vi "CalculateDatagram.vi"(0 "mqttCmd in":refnum<class "BaseMqttMsg.lvclass">, 5 "FixedHeaderByte1":u8 format="%08b", 7 "variableHeader":u8[](array[numeric]), 9 "payload":u8[](array[numeric]), 11 "error in (no error)":errorcluster) -> (4 "mqttCmd out":refnum<class "BaseMqttMsg.lvclass">, 6 "Datagram":u8[](array[numeric]), 15 "error out":errorcluster)   [LabVIEW 2020, in "BaseMqttMsg.lvclass"]
uses:
  BaseMqttMsg.lvclass
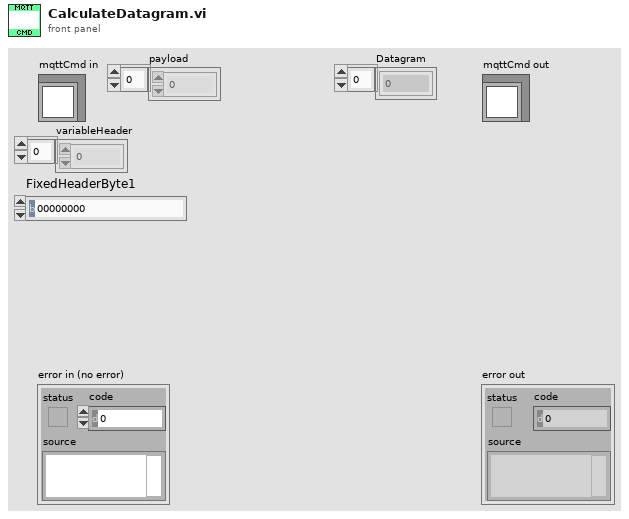
[diagram p1: front panel]
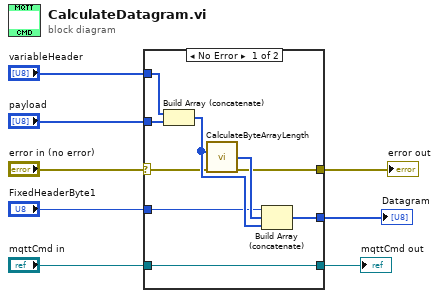
[diagram p0: block diagram]
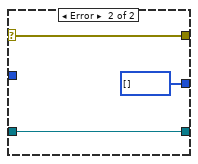
[diagram p2: hidden frame]
diagram:
  n1 = case shown="No Error" "error in (no error)" {
    selector: "error in (no error)" -> [w11 w20]
    tunnel: [w10 w20] -> w7
    tunnel: [w17 w19] -> w5
    tunnel: "mqttCmd in" -> [w17 w19]
    tunnel: "variableHeader" -> [w14 _]
    tunnel: "payload" -> [w13 _]
    tunnel: "FixedHeaderByte1" -> [w12 _]
    tunnel: [w9 u8[] []] -> w1
    frame No Error {
      n2 = Build Array (concatenate)(w14, w13) -> (w16:u8[])
      n3 = call "CalculateByteArrayLength.vi"("byteArry in"=w16, "error in (no error)"=w11) -> ("length out"=w15:u8[], "error out"=w10:errorcluster)  [unwired: 12 in]
      n4 = Build Array (concatenate)(w12, w15, w16) -> (w9:u8[])
    }
    frame Error {
    }
  }
  "error out" <- w7
  "mqttCmd out" <- w5
  "Datagram" <- w1
